vi "grab image.vi"(8 "error in (no error)":errorcluster, 10 "Image In":T1, 11 "Camera":T2) -> (0 "error out":errorcluster, 2 "Image Out":T1, 3 "Camera out":T2)   [LabVIEW 2022 SP3, in "Vision.lvlib"]
uses:
  Vision.lvlib
  camera.ctl
  camera driver.ctl
  <vilib>/vision/Image Controls.llb/IMAQ Image.ctl
  C:/Users/Caleb/Desktop/nebraska-silicon-lab/pixel-gantry-extra/LV/bin/uEyeDotNet.dll
  bin/uEyeDotNet.dll
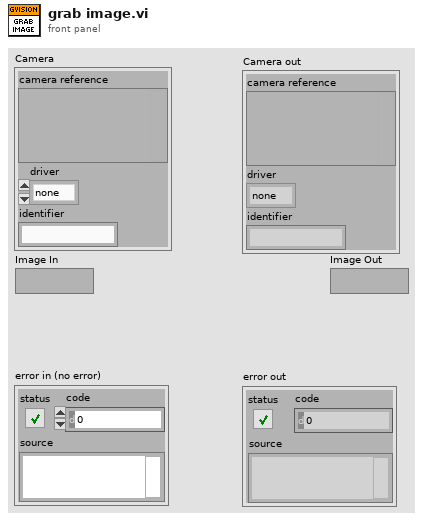
[diagram p1: front panel]
types:
  T1 = typedef "IMAQ Image.ctl" = refnum<image>
  T2 = typedef "Vision.lvlib/camera.ctl" = cluster{"camera reference":variant, "driver":T3, "identifier":string}
  T3 = typedef "Vision.lvlib/camera driver.ctl" = enum16{"none", "ueye", "wmf"}
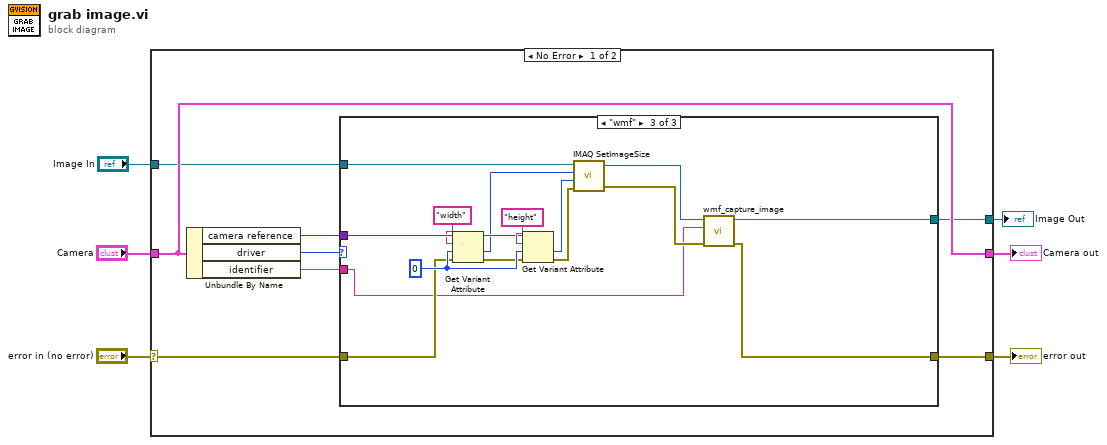
[diagram p0: block diagram]
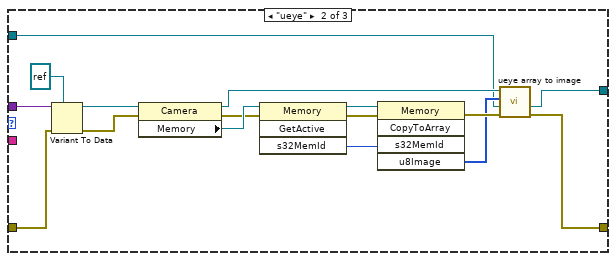
[diagram p3: hidden frame]
diagram:
  n1 = case shown="No Error" "error in (no error)" {
    selector: "error in (no error)" -> [w7 w49]
    tunnel: [w11 w49] -> w5
    tunnel: "Camera" -> [w10 w48]
    tunnel: [w10 w48] -> w3
    tunnel: [w9 _] -> w2
    tunnel: "Image In" -> [w8 _]
    frame No Error {
      n2 = Unbundle By Name(w10) -> ("camera reference"=w13:variant, "driver"=w14:T3, "identifier"=w12:string)
      n3 = case shown="\"wmf\"" w14 {
        tunnel: w13 -> [_ w26 w47]
        tunnel: w12 -> [_ _ w32]
        tunnel: w7 -> [w15 w23 w41]
        tunnel: [w15 w18 w33] -> w11
        tunnel: w8 -> [_ w17 w40]
        tunnel: [_ w16 w35] -> w9
        frame "none" {
        }
        frame "ueye" {
          n4 = Variant To Data(error in=w23, type=refnum<k24> refnum ("reference"), Variant=w26) -> (data=w24:refnum<k24>, error out=w22:errorcluster)
          n5 = property class="Camera"(reference=w24, error in=w22) -> (reference out=w21:refnum<k24>, error out=w30:errorcluster, "Memory"=w31:refnum<k24>)
          n6 = invoke class="Memory" method="GetActive"(reference=w31, error in=w30) -> (reference out=w27:refnum<k24>, error out=w28:errorcluster, "s32MemId"=w29:i32)  [unwired: 2 in, 1 out]
          n7 = invoke class="Memory" method="CopyToArray"(reference=w27, error in=w28, "s32MemId"=w29) -> (error out=w20:errorcluster, "u8Image"=w19:u8[])  [unwired: 2 in, 3 out]
          n8 = call "ueye array to image.vi"("Error In"=w20, "Image In"=w17, "InArray"=w19, "Camera Reference"=w21) -> ("Error Out"=w18:errorcluster, "Image Out"=w16:T1)  [unwired: 5 in, 1 out]
        }
        frame "wmf" {
          w43 = 0
          n9 = Get Variant Attribute(Variant=w47, name="width", default value (empty Variant)=w43, error in=w41) -> (duplicate Variant=w44:variant, value=w39:i32, error out=w42:errorcluster)  [unwired: 1 out]
          n10 = Get Variant Attribute(Variant=w44, name="height", default value (empty Variant)=w43, error in=w42) -> (value=w38:i32, error out=w37:errorcluster)  [unwired: 2 out]
          n11 = call "IMAQ SetImageSize"("error in (no error)"=w37, "Y Resolution"=w38, "X Resolution"=w39, "Image"=w40) -> ("error out"=w34:errorcluster, "Image Out"=w36:T1)  [unwired: 1 in]
          n12 = call "wmf_capture_image.vi"("error in (no error)"=w34, "identifier"=w32, "Image in"=w36) -> ("error out"=w33:errorcluster, "Image out"=w35:T1)  [unwired: 7 in]
        }
      }
    }
    frame Error {
    }
  }
  "error out" <- w5
  "Camera out" <- w3
  "Image Out" <- w2
